vi "UI elements.vi"() -> ()   [LabVIEW 2025]
uses:
  <vilib>/userDefined/Silver/nirio_resource_slv.ctl
  <vilib>/userDefined/High Color/nirio_resource_hc.ctl
panel:
  out "BOOLEAN 6":bool
  out "BOOLEAN 5":bool
  out "BOOLEAN 4":bool
  out "BOOLEAN 3":bool
  out "BOOLEAN 2":bool
  in  "ENUM 4":enum16{"ITEM0"}(ring)
  in  "RING 4":u16(ring) items=["TERMINATION OFF", "TERMINATION ON"]
  in  "ENUM 3":enum16{"ITEM0"}(ring)
  in  "RING 3":u16(ring) items=["TERMINATION OFF", "TERMINATION ON"]
  in  "ENUM 2":enum16{"ITEM0"}(ring)
  out "PATH TO CONFIG 5":path
  out "PATH TO CONFIG 4":path
  in  "PATH TO CONFIG 3":path
  in  "PATH TO CONFIG 2":path
  in  "XNET DEVICE 2":refnum<k21>
  in  "SWITCH DEVICE 2":refnum<k15>
  in  "RIO DEVICE 2":T1
  in  "STOP 4":bool
  in  "START 2":bool
  in  "STOP 3":bool
  in  "BUTTON 2":bool
  in  "OK":bool
  in  "SETTINGS":enum32{"SETTING1", "SETTING2"}(tab)
  in  "BOOL ARRAY - GREY":bool[][](array[boolean])
  in  "BOOL ARRAY":bool[][](array[boolean])
  in  "SETTINGS":bool
  out "ERROR":bool
  in  "SETTINGS":bool
  in  "INFO":bool
  in  "REMOVE":bool
  in  "MOVE UP":bool
  in  "MOVE DOWN":bool
  in  "ADD":bool
  in  "STOP 2":bool
  out "RESULT":bool
  out "RESULT":bool
  in  "RING 2":u16(ring) items=["TERMINATION OFF", "TERMINATION ON"]
  out "STATUS":bool
  in  "COMBO BOX  LONG":string(combo)
  out "ARRAY - STRING":string[](array[string])
  in  "ARRAY - STRING":string[](array[string])
  out "ARRAY - NUMERIC":dbl[](array[numeric])
  in  "ARRAY - NUMERIC":dbl[](array[numeric])
  out "PATH TO CONFIG - SHORT":path
  out "PATH TO CONFIG":path
  in  "PATH TO CONFIG - SHORT":path
  out "STATE MESSAGE 2":string
  in  "STATE MESSAGE":string
  out "LONG STRING":string
  in  "LONG STRING":string
  out "MID STRING":string
  in  "MID STRING":string
  in  "START":bool
  in  "ENUM":enum16{"ITEM0"}(ring)
  in  "RING":u16(ring) items=["ITEM0"]
  out "ERROR":errorcluster
  in  "PATH TO CONFIG":path
  in  "COMBO BOX":string(combo)
  out "SHORT STRING":string
  in  "SHORT STRING":string
  in  "RADIO BUTTON":enum32{"Item 0", "Item 1"}(radio)
  in  "CHECKBOX":bool
  out "BOOLEAN":bool
  in  "STOP":bool
  in  "BUTTON":bool
  out "NUMERIC":dbl
  in  "NUMERIC":dbl
  in  "XNET DEVICE":refnum<k21>
  in  "SWITCH DEVICE":refnum<k15>
  in  "SWITCH DEVICE":refnum<k15>
  in  "SWITCH DEVICE":refnum<k15>
  in  "RIO DEVICE":T1
  in  "RIO DEVICE":T2
  out "DISPLAY":T3(plugin-control)
  # "font 14"
  # "FONT 14"
  # "font 15"
  # "FONT 15"
  # "looks not good but alingned with grid"
  # "InstrumentStudio style guide colors\nRED _        NIErrorBrush \t\t#C42126\nORANGE  NIWarningBrush \t\t#FF8900\nGREEN      NISuccessBrush \t\t#20B25B\nBLUE         NIProbeBrush \t\t#006A93\n?                 NIGuidelineBrush \t\t#FC9500\nGrey           NIButtonFillBrush \t\t#E9EBEC (Offset: 0%)\n                                                      #D9DEE1 (Offset: 40%)\n\nrecommended sizes for well alignment\n24\n\n48\n\n72\n\n96\n\n120\n\n144\n\n168\n\n192\n\n216\n\n240"
  # "small button"
  # "large button"
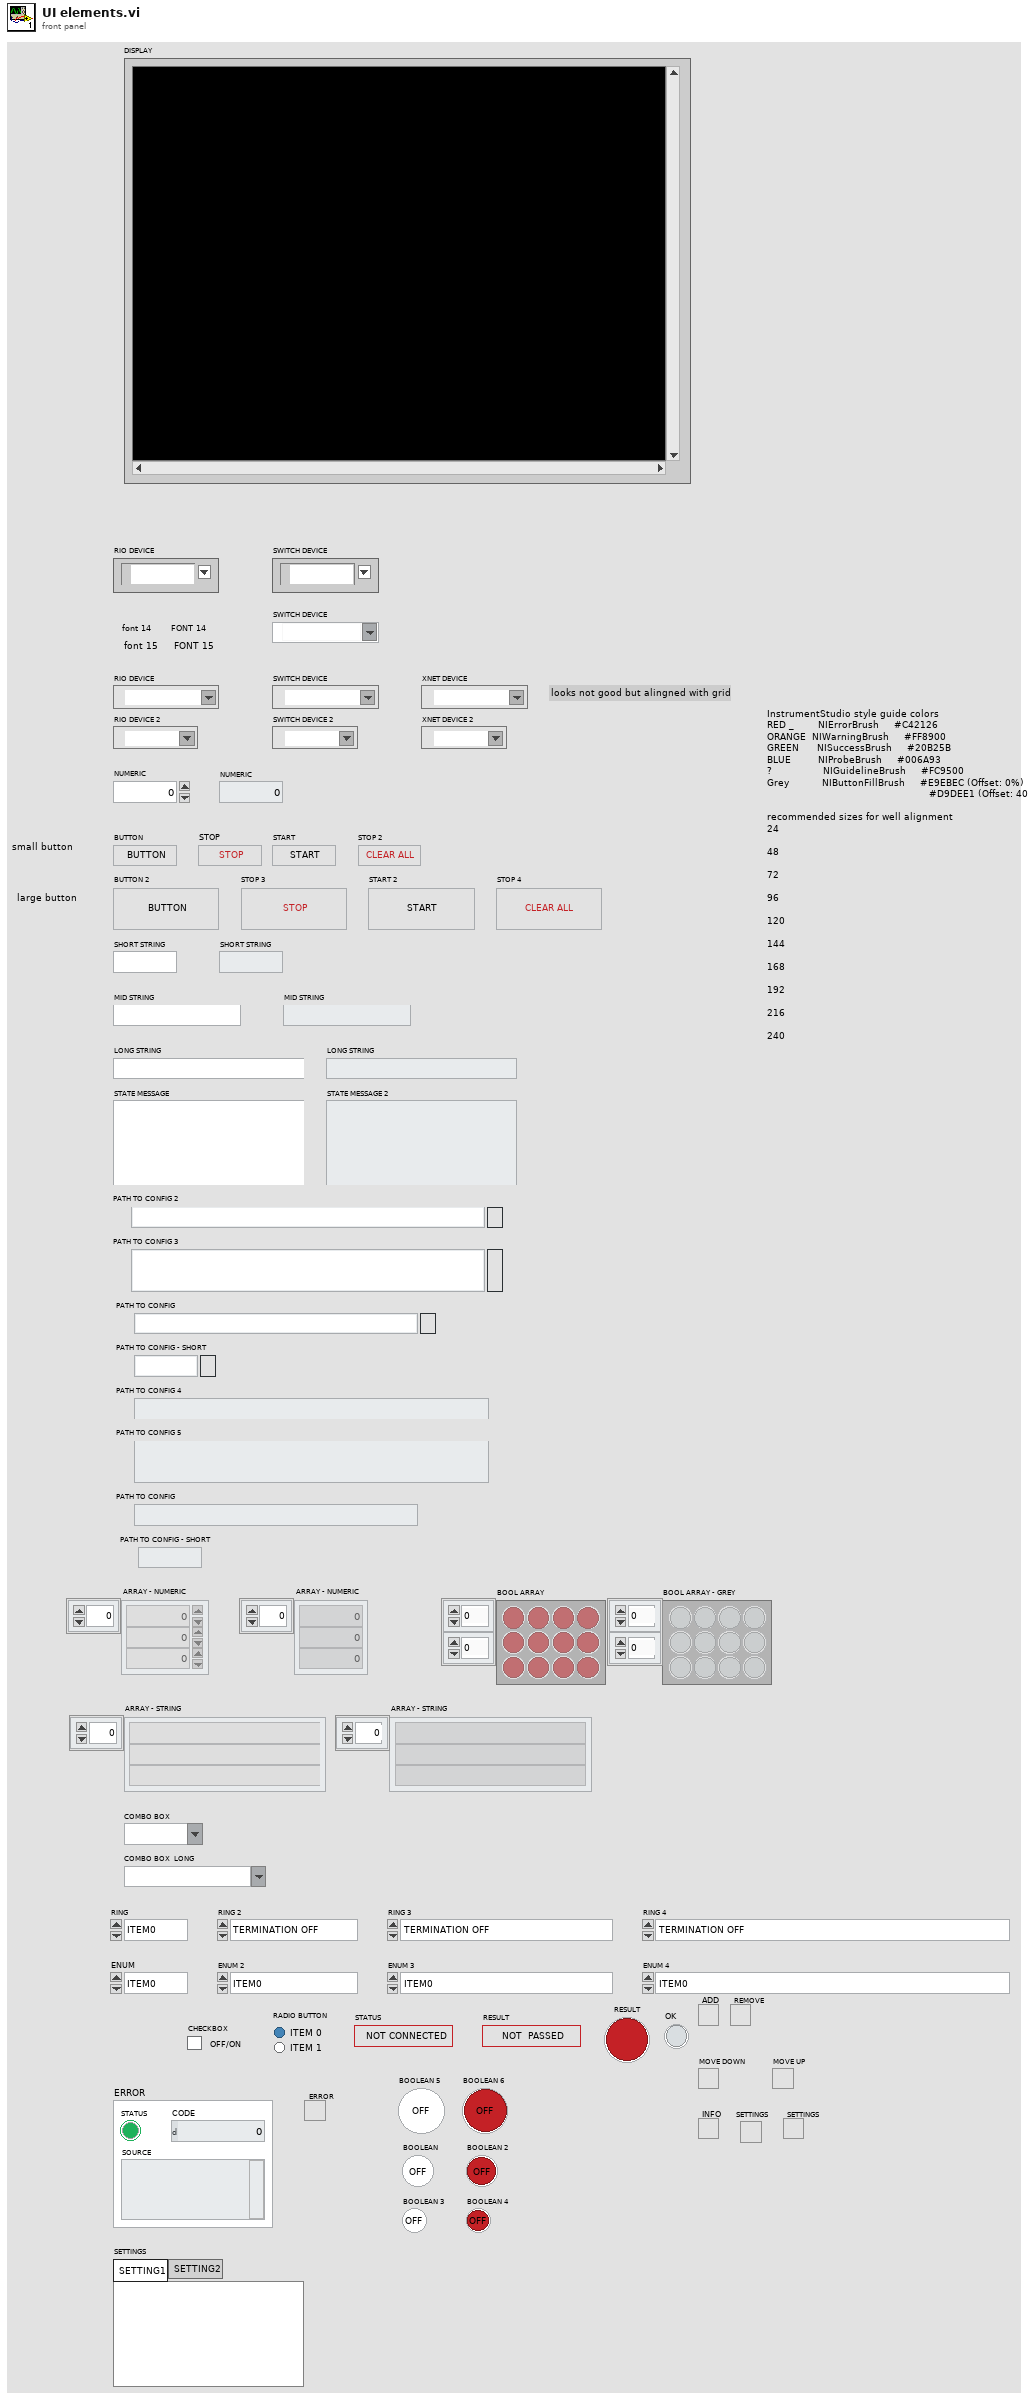
[diagram p1: front panel]
types:
  T1 = typedef "nirio_resource_hc.ctl" = tag
  T2 = typedef "nirio_resource_slv.ctl" = tag
  T3 = typedef "IMAQ Image.ctl" = refnum<image>
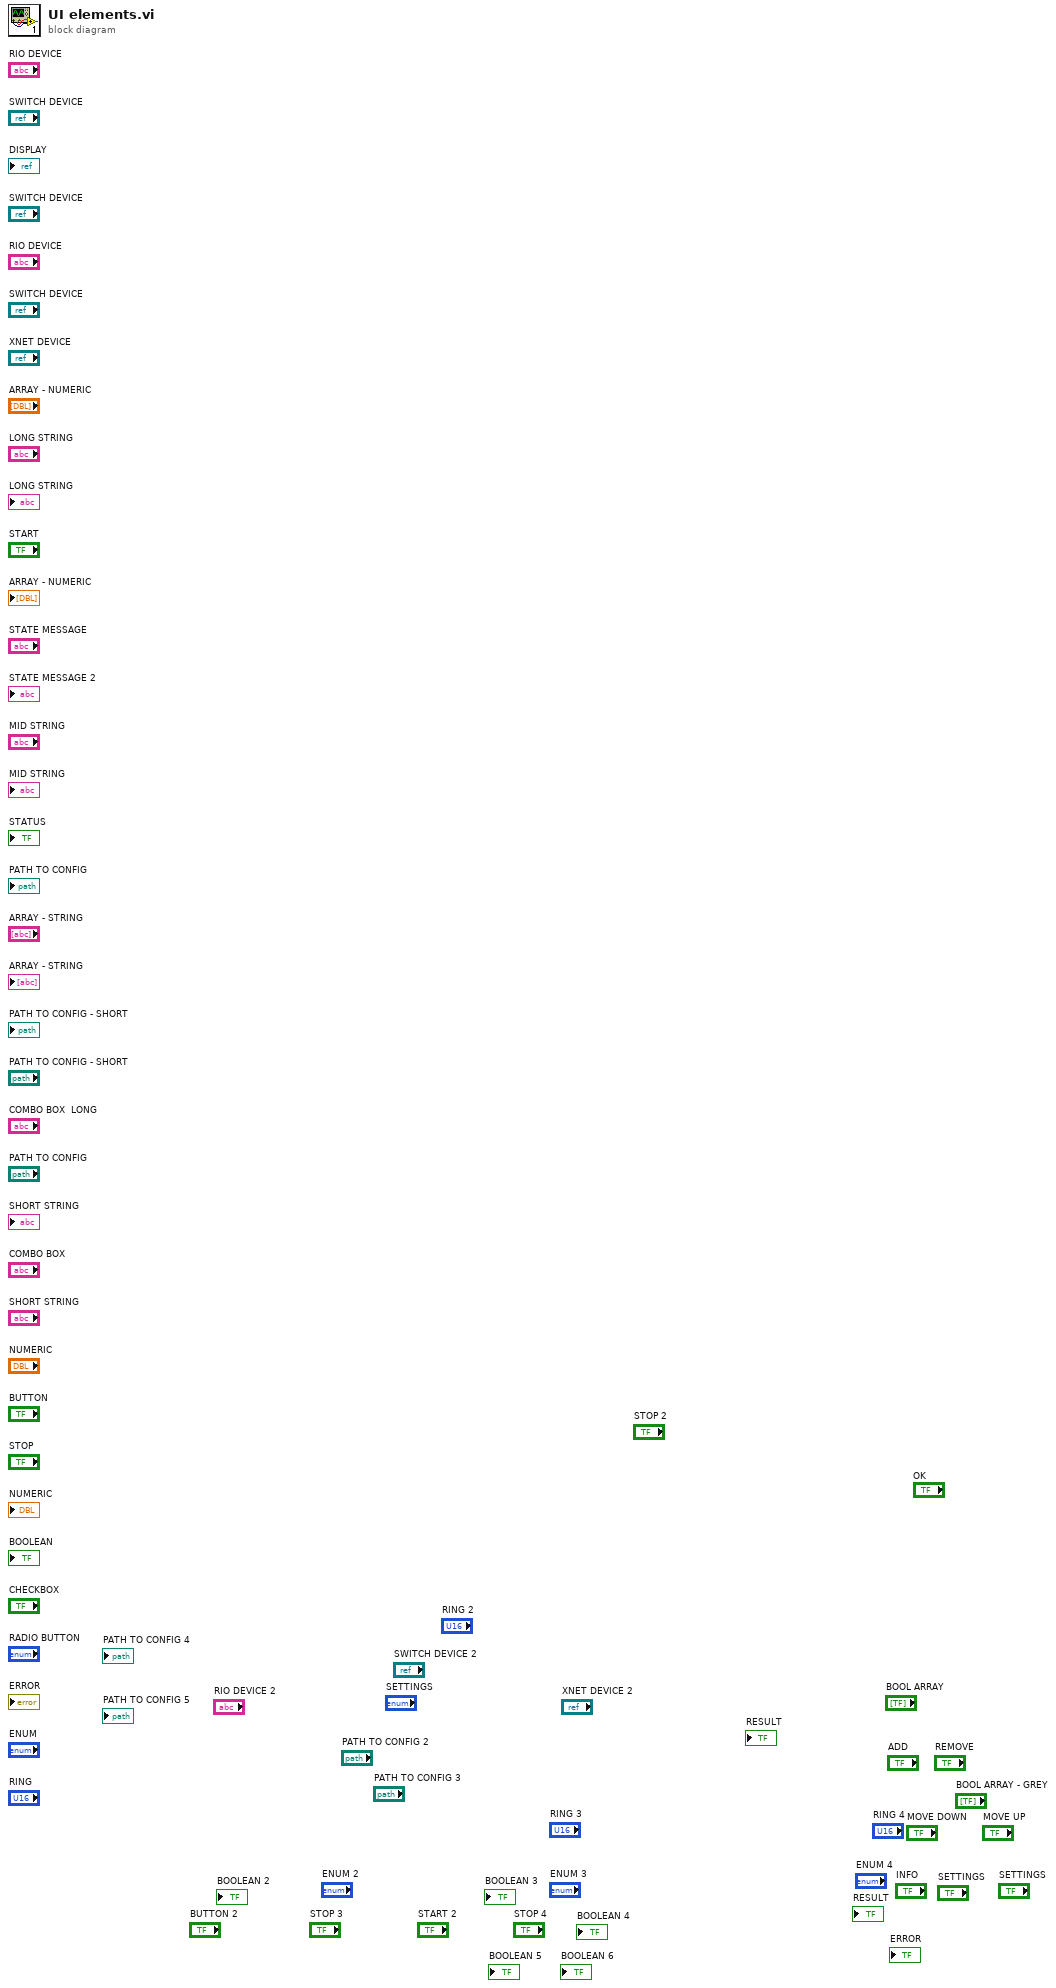
[diagram p0: block diagram]
diagram:
